vi "create basic config.vi"(8 "error in":errorcluster) -> (0 "error out":errorcluster, 1 "instance identifier":string, 2 "generated channels":refnum<class "TBM channel.lvclass">[](array[class]), 3 "user tag bus module configuration out":refnum<class "user tag bus module configuration.lvclass">)   [LabVIEW 2013, in "user code tests.lvlib"]
uses:
  user code tests.lvlib
  module/configuration/user tag bus module configuration.lvclass
  <vilib>/NI/Tag Bus Module Framework/channel/TBM channel.lvclass
  <vilib>/NI/Tag Bus Module Framework/root configuration/TBM configuration.lvclass/TBM configuration.ctl
  module/configuration/gains.ctl
  <vilib>/NI/Tag Bus Module Framework/root configuration/Read instance name.vi
  <vilib>/NI/Tag Bus Module Framework/root configuration/create GUID.vi
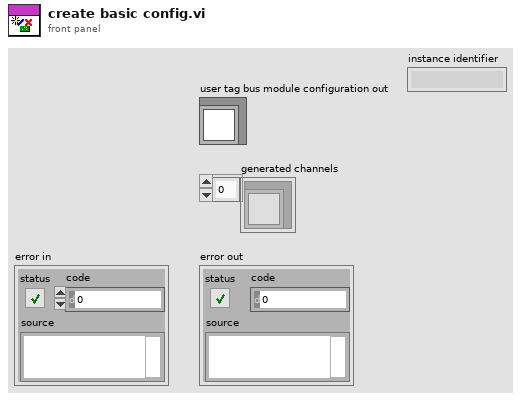
[diagram p1: front panel]
types:
  T1 = typedef "user tag bus module configuration.lvclass/gains.ctl" = cluster{"Kp":dbl, "Ki":dbl, "Kd":dbl}
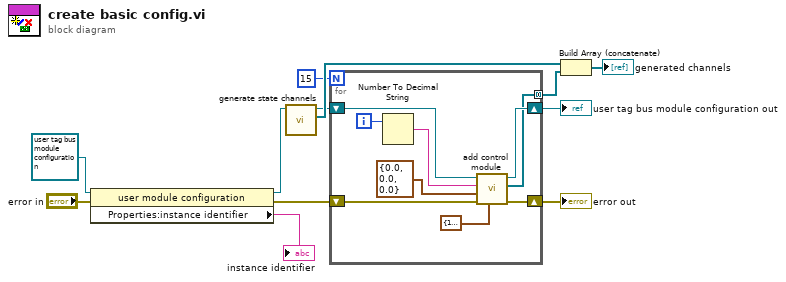
[diagram p0: block diagram]
diagram:
  n1 = property class="user module configuration"(reference=refnum<class "user tag bus module configuration.lvclass"> refnum ("tag bus configurable plugin module configuration"), error in="error in") -> (reference out=w4:refnum<class "user tag bus module configuration.lvclass">, error out=w2:errorcluster, "Properties:instance identifier"=→"instance identifier":string)
  n2 = call "generate state channels.vi"("tag bus configurable plugin module configuration in"=w4) -> ("generated channels"=w8:refnum<class "TBM channel.lvclass">[], "tag bus configurable plugin module configuration out"=w7:refnum<class "user tag bus module configuration.lvclass">)  [unwired: 9 in]
  n3 = for {
    N: 15 -> [_]
    shift-right: [w20] -> w11
    shift-left: w7 -> [w21]
    tunnel: [w19] -> w9 mode=concatenating
    shift-right: [w14] -> w12
    shift-left: w2 -> [w13]
    i -> [w16]
    n4 = Number To Decimal String(number=w16) -> (decimal integer string=w15:string)  [unwired: 1 in]
    n5 = call "add control module.vi"("output range"=cluster{"output high":dbl, "output low":dbl} {"output high"=100.0, "output low"=-100.0}, "error in"=w13, "gains"=T1 {"Kp"=0.0, "Ki"=0.0, "Kd"=0.0}, "name"=w15, "user module configuration in"=w21) -> ("error out"=w14:errorcluster, "generated channels"=w19:refnum<class "TBM channel.lvclass">[], "user module configuration out"=w20:refnum<class "user tag bus module configuration.lvclass">)  [unwired: 3 in, 1 out]
  }
  "error out" <- w12
  "user tag bus module configuration out" <- w11
  n6 = Build Array (concatenate)(w8, w9) -> (→"generated channels":refnum<class "TBM channel.lvclass">[])
